vi "LoadMasks.vi"(10 "url":string, 11 "ComboBox in":refnum<vi>) -> (0 "error out":errorcluster)   [LabVIEW 2020]
uses:
  <vilib>/httpClient/LabVIEWHTTPClient.lvlib
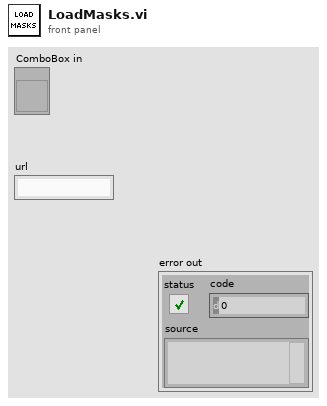
[diagram p1: front panel]
types:
  T1 = typedef "LabVIEWHTTPClient.lvlib/ClientHandle.ctl" = refnum<k1>
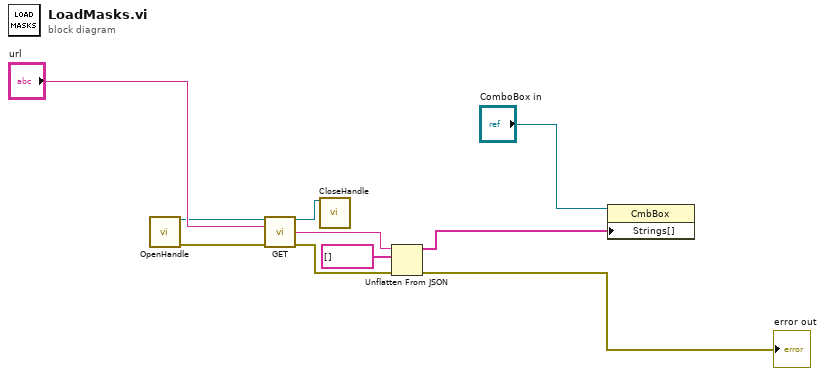
[diagram p0: block diagram]
diagram:
  n1 = call <vilib>:"OpenHandle.vi"() -> ("client handle out"=w1:T1, "error out"=w10:errorcluster)  [unwired: 14 in]
  n2 = call <vilib>:"GET.vi"("client handle"=w1, "url"="url", "error in (no error)"=w10) -> ("client handle out"=w2:T1, "body"=w3:string, "error out"=w9:errorcluster)  [unwired: 9 in, 1 out]
  n3 = call <vilib>:"CloseHandle.vi"("client handle"=w2) -> ()  [unwired: 14 in, 1 out]
  n4 = Unflatten From JSON(JSON string=w3, type and defaults=string[] [], error in (no error)=w9) -> (value=w7:string[], error out=→"error out":errorcluster)  [unwired: 4 in]
  n5 = property class="CmbBox"(reference="ComboBox in", "Strings[]"=w7) -> ()  [unwired: 1 in, 2 out]
